vi "Rec Get Column Properties (R).vi"(4 "error in (no error)":errorcluster, 6 "column index":variant, 7 "recordset reference":T3) -> (0 "error out":errorcluster, 1 "column properties":T1, 3 "recordset reference out":T3)   [LabVIEW 2017, in "NI_Database_API.lvlib"]
doc: "Gets properties of the object as determined by the inputs. This VI works for connections, commands, recordsets, columns, and parameters. Wire data to the reference input to determine the polymorphic instance to use or manually select the instance."
uses:
  <vilib>/addons/database/NI_Database_API.lvlib
  <vilib>/addons/database/Recordset.llb/Rec ObjectReference.ctl
  <vilib>/addons/database/Recordset.llb/Rec Column Properties.ctl
  <vilib>/addons/database/Auxilliary.llb/DB Tools DataTypes.ctl
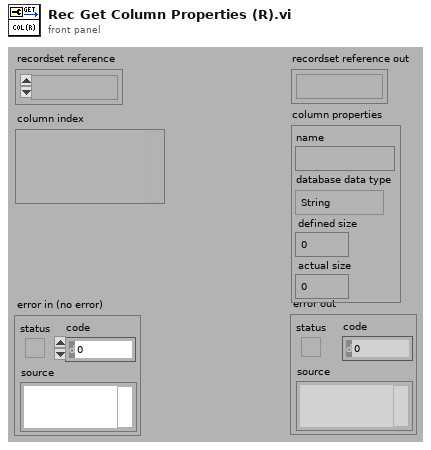
[diagram p1: front panel]
types:
  T1 = typedef "NI_Database_API.lvlib/Rec Column Properties.ctl" = cluster{"name":string, "database data type":T2, "defined size":i32, "actual size":i32}
  T2 = typedef "NI_Database_API.lvlib/DB Tools DataTypes.ctl" = enum16{"String", "Long (I32)", "Single (SGL)", "Double (DBL)", "Date/Time", "Binary"}
  T3 = typedef "NI_Database_API.lvlib/Rec ObjectReference.ctl" = refnum<k1>
  T4 = typedef "NI_Database_API.lvlib/Rec Properties.ctl" = cluster{"column count":i32, "record index":i32, "record count":i32, "bof?":bool, "eof?":bool, "cursor type":T5, "cache size":i32, "state":enum16{"closed", "open"}}
  T5 = typedef "NI_Database_API.lvlib/DB Tools Cursor Type.ctl" = enum16{"forward-only", "keyset", "dynamic", "static"}
  T6 = typedef "NI_Database_API.lvlib/Rec DataMembers.ctl" = cluster{"ADODB._Recordset":refnum<k7>, "Connection":T7}
  T7 = typedef "NI_Database_API.lvlib/Conn ObjectReference.ctl" = refnum<k1>
  T8 = cluster{"Name":string, "data type":T2, "DefinedSize":i32, "ActualSize":i32}
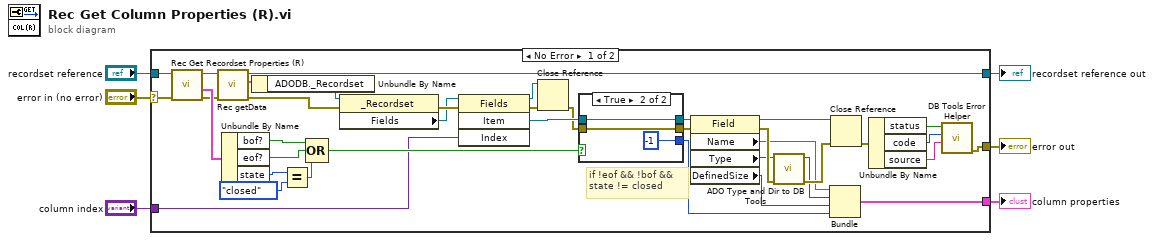
[diagram p0: block diagram]
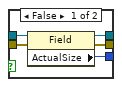
[diagram p2: hidden frame]
diagram:
  n1 = case shown="No Error" "error in (no error)" {
    selector: "error in (no error)" -> [w8 w54]
    tunnel: "recordset reference" -> [w44 w53]
    tunnel: [w23 w53] -> w5
    tunnel: "column index" -> [w18 _]
    tunnel: [w14 _] -> w3
    tunnel: [w9 w54] -> w2
    frame No Error {
      # "if !eof && !bof &&\nstate != closed"
      n2 = call <vilib>:"Rec Get Recordset Properties (R).vi"("error in (no error)"=w8, "recordset reference"=w44) -> ("error out"=w17:errorcluster, "recordset properties"=w42:T4, "recordset reference out"=w19:T3)  [unwired: 3 out]
      n3 = call <vilib>:"Rec getData.vi"("error in (no error)"=w17, "recordset reference"=w19) -> ("error out"=w25:errorcluster, "data"=w20:T6, "recordset reference out"=w23:T3)  [unwired: 3 out]
      n4 = Unbundle By Name(w42) -> ("bof?"=w35:bool, "eof?"=w43:bool, "state"=w37:enum16{"closed", "open"})
      n5 = Unbundle By Name(w20) -> ("ADODB._Recordset"=w24:refnum<k7>)
      n6 = Equal?(x=w37, y=enum16{"closed", "open"}."closed" ("state")) -> (x = y?=w34:bool)
      n7 = Compound Arithmetic op=OR(w35, w43, w34) -> (w38:bool)
      n8 = property class="_Recordset"(reference=w24, error in=w25) -> (error out=w26:errorcluster, "Fields"=w7:refnum<k7>)  [unwired: 1 out]
      n9 = invoke class="Fields" method="Item"(reference=w7, error in=w26, "Index"=w18) -> (reference out=w21:refnum<k7>, error out=w22:errorcluster, "Item"=w16:refnum<k7>)  [unwired: 1 in, 1 out]
      n10 = Close Reference(reference=w21, error in (no error)=w22) -> (error out=w15:errorcluster)
      n11 = case shown="True" w38 {
        tunnel: [w48 w52] -> w40
        tunnel: w16 -> [w46 w52]
        tunnel: w15 -> [w49 w51]
        tunnel: [w47 w51] -> w39
        tunnel: [w45 -1 ("ActualSize")] -> w27
        frame False {
          n12 = property class="Field"(reference=w46, error in=w49) -> (reference out=w48:refnum<k7>, error out=w47:errorcluster, "ActualSize"=w45:i32)
        }
        frame True {
        }
      }
      n13 = property class="Field"(reference=w40, error in=w39) -> (reference out=w33:refnum<k7>, error out=w41:errorcluster, "Name"=w31:string, "Type"=w30:i32, "DefinedSize"=w28:i32)
      n14 = call <vilib>:"ADO Type and Dir to DB Tools.vi"("error in (no error)"=w41, "ADO type"=w30) -> ("error out"=w32:errorcluster, "data type"=w29:T2)  [unwired: 1 in, 3 out]
      n15 = Bundle("Name"=w31, "data type"=w29, "DefinedSize"=w28, "ActualSize"=w27) -> (w14:T8)  [unwired: 1 out]
      n16 = Close Reference(reference=w33, error in (no error)=w32) -> (error out=w10:errorcluster)
      n17 = Unbundle By Name(w10) -> ("status"=w12:bool, "code"=w11:i32, "source"=w13:string)
      n18 = call <vilib>:"DB Tools Error Helper.vi"("source"=w13, "code"=w11, "status"=w12) -> ("error out"=w9:errorcluster)  [unwired: 1 in, 7 out]
    }
    frame Error {
    }
  }
  "recordset reference out" <- w5
  "error out" <- w2
  "column properties" <- w3
